vi "interpolate.vi"(10 "compensation parameters in":T1, 11 "State in":T2={"control refs"={"z offset"=refnum, "laser intensity"=refnum, "XY graph"=refnum}, "error"={"status"=FALSE, "code"=0, "source"=""}, "free-run?"=TRUE, "range (um)"=400, "interpolate?"=FALSE, "settings"={"fix points"=[], "compensation parameters"={"A"=0.0, "lambda"=0.0, "C"=0.0}}} caption="State") -> (2 "compensation parameters out":T1, 3 "State out":T2={"control refs"={"z offset"=refnum, "laser intensity"=refnum, "XY graph"=refnum}, "error"={"status"=FALSE, "code"=0, "source"=""}, "free-run?"=TRUE, "range (um)"=400, "interpolate?"=FALSE, "settings"={"fix points"=[], "compensation parameters"={"A"=0.0, "lambda"=0.0, "C"=0.0}}} caption="State")   [LabVIEW 2010, in "XIntensityCompensation.xctl"]
uses:
  XIntensityCompensation.xctl
  state.ctl
  control_refs.ctl
  settings_cluster.ctl
  data.ctl
  <vilib>/Analysis/6fits.llb/Curve Fitting Criteria.ctl
  <vilib>/Analysis/NI_AALPro.lvlib
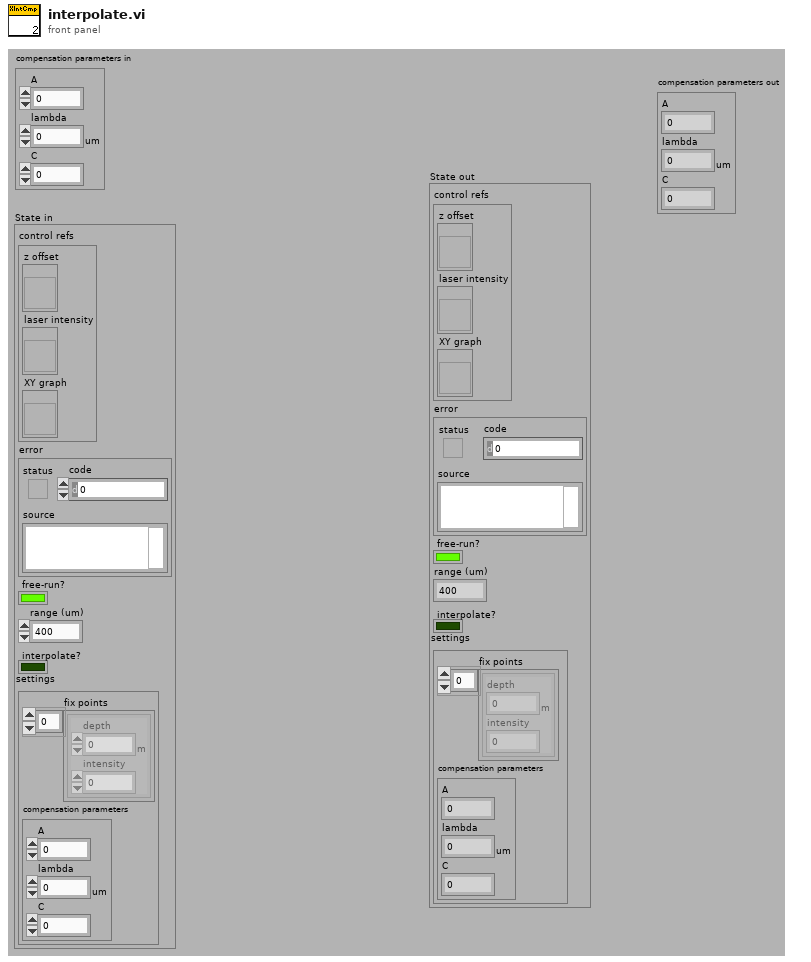
[diagram p1: front panel]
types:
  T1 = typedef "XIntensityCompensation.xctl/data.ctl" = cluster{"A":dbl, "lambda":dbl[unit], "C":dbl}
  T2 = typedef "XIntensityCompensation.xctl/state.ctl" = cluster{"control refs":T3, "error":errorcluster, "free-run?":bool, "range (um)":i32, "interpolate?":bool, "settings":T4}
  T3 = typedef "XIntensityCompensation.xctl/control_refs.ctl" = cluster{"z offset":refnum<vi>, "laser intensity":refnum<vi>, "XY graph":refnum<vi>}
  T4 = typedef "XIntensityCompensation.xctl/settings_cluster.ctl" = cluster{"fix points":cluster{"depth":dbl[unit], "intensity":dbl}[], "compensation parameters":T1}
  T5 = typedef "NI_AALPro.lvlib/Curve Fitting Criteria.ctl" = u16
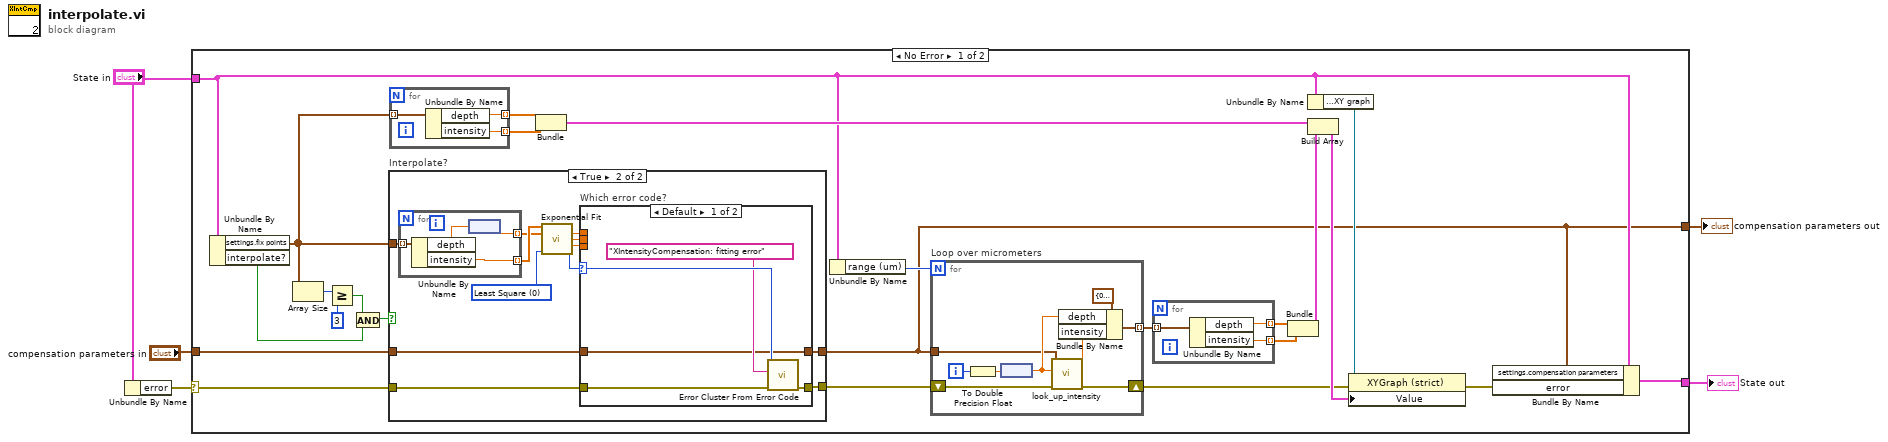
[diagram p0: block diagram]
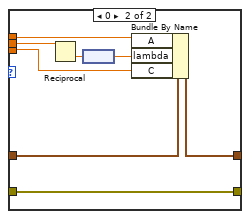
[diagram p3: hidden frame]
diagram:
  n1 = Unbundle By Name("State in") -> ("error"=w5:errorcluster)
  n2 = case shown="No Error" w5 {
    selector: w5 -> [w21 _]
    tunnel: "State in" -> [w11 w77]
    tunnel: [w19 w77] -> w3
    tunnel: "compensation parameters in" -> [w10 w76]
    tunnel: [w6 w76] -> w1
    frame No Error {
      n3 = Unbundle By Name(w11) -> ("settings.fix points"=w17:cluster{"depth":dbl[unit], "intensity":dbl}[], "interpolate?"=w13:bool)
      n4 = Array Size(array=w17) -> (size(s)=w16:i32)
      n5 = Greater Or Equal?(x=w16, y=3) -> (x >= y?=w14:bool)
      n6 = And(x=w14, y=w13) -> (x .and. y?=w12:bool)
      n7 = case "Interpolate?" shown="True" w12 {
        tunnel: w17 -> [_ w43]
        tunnel: w21 -> [w31 w42]
        tunnel: [w31 w41] -> w8
        tunnel: w10 -> [w30 w33]
        tunnel: [w30 w32] -> w6
        frame False {
        }
        frame True {
          w38 = T5 0 items=["Least Square", "Least Absolute Residual", "Bisquare"] ("method")
          n8 = for {
            tunnel: w43 -> [w60] mode=indexing
            tunnel: [w59] -> w40 mode=indexing
            tunnel: [w58] -> w39 mode=indexing
            n9 = Unbundle By Name(w60) -> ("depth"=w57:dbl[unit], "intensity"=w59:dbl)
            n10 = node(w57) -> (w58:dbl)
          }
          n11 = call <vilib>:"Exponential Fit.vi"("Y"=w40, "X"=w39, "method"=w38) -> ("amplitude"=w36:dbl, "damping"=w35:dbl, "offset"=w37:dbl, "error"=w34:i32)  [unwired: 7 in, 2 out]
          n12 = case "Which error code?" shown="Default" w34 {
            selector: w34 -> [w48 _]
            tunnel: w37 -> [_ w54]
            tunnel: w36 -> [_ w55]
            tunnel: w35 -> [_ w53]
            tunnel: w42 -> [w47 w56]
            tunnel: [w45 w56] -> w41
            tunnel: w33 -> [w44 w52]
            tunnel: [w44 w49] -> w32
            frame Default {
              n13 = call <vilib>:"Error Cluster From Error Code.vi"("error in (no error)"=w47, "error message (\"\")"="XIntensityCompensation: fitting error" ("error message (\"\")"), "error code (0)"=w48) -> ("error out"=w45:errorcluster)  [unwired: 6 in]
            }
            frame 0 {
              n14 = Reciprocal(x=w53) -> (1/x=w50:dbl)
              n15 = node(w50) -> (w51:dbl[unit])
              n16 = Bundle By Name(cluster=w52, "A"=w55, "lambda"=w51, "C"=w54) -> (w49:T1)
            }
          }
        }
      }
      n17 = for {
        tunnel: w17 -> [w75] mode=indexing
        tunnel: [w73] -> w29 mode=indexing
        tunnel: [w74] -> w26 mode=indexing
        n18 = Unbundle By Name(w75) -> ("depth"=w73:dbl[unit], "intensity"=w74:dbl)
      }
      n19 = Bundle(w29, w26) -> (w25:cluster{dbl[unit][], dbl[]})  [unwired: 1 in]
      n20 = Unbundle By Name(w11) -> ("range (um)"=w18:i32)
      n21 = for "Loop over micrometers" {
        N: w18 -> [_]
        tunnel: [w68] -> w9 mode=indexing
        shift-right: [w62] -> w7
        shift-left: w8 -> [w65]
        tunnel: w6 -> [w61]
        i -> [w67]
        n22 = To Double Precision Float(number=w67) -> (double precision float=w66:dbl)
        n23 = node(w66) -> (w64:dbl[unit])
        n24 = call "look_up_intensity.vi"("error in (no error)"=w65, "z offset"=w64, "compensation parameters"=w61) -> ("error out"=w62:errorcluster, "intensity"=w63:dbl)  [unwired: 7 in]
        n25 = Bundle By Name(cluster=cluster{"depth":dbl[unit], "intensity":dbl} {"depth"=0.0, "intensity"=0.0} ("intensity/depth combination"), "depth"=w64, "intensity"=w63) -> (w68:cluster{"depth":dbl[unit], "intensity":dbl})
      }
      n26 = for {
        tunnel: w9 -> [w72] mode=indexing
        tunnel: [w71] -> w28 mode=indexing
        tunnel: [w70] -> w27 mode=indexing
        n27 = Unbundle By Name(w72) -> ("depth"=w71:dbl[unit], "intensity"=w70:dbl)
      }
      n28 = Bundle(w28, w27) -> (w23:cluster{dbl[unit][], dbl[]})  [unwired: 1 in]
      n29 = Unbundle By Name(w11) -> ("control refs.XY graph"=w24:refnum<vi>)
      n30 = Build Array(w25, w23) -> (w22:cluster{dbl[unit][], dbl[]}[])
      n31 = property class="XYGraph (strict)"(reference=w24, error in=w7, "Value"=w22) -> (error out=w20:errorcluster)  [unwired: 1 out]
      n32 = Bundle By Name(cluster=w11, "settings.compensation parameters"=w6, "error"=w20) -> (w19:T2)
    }
    frame Error {
    }
  }
  "State out" <- w3
  "compensation parameters out" <- w1
